vi "multiColorWormMolecule.vi"(0 "molecule":string) -> (1 "slider position":i32, 2 "filter wheel position":i32)   [LabVIEW 2017]
panel:
  # "Returns indexes of filter wheel and slider/shutter position\ngiven the molecule."
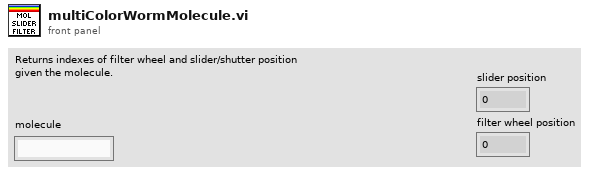
[diagram p1: front panel]
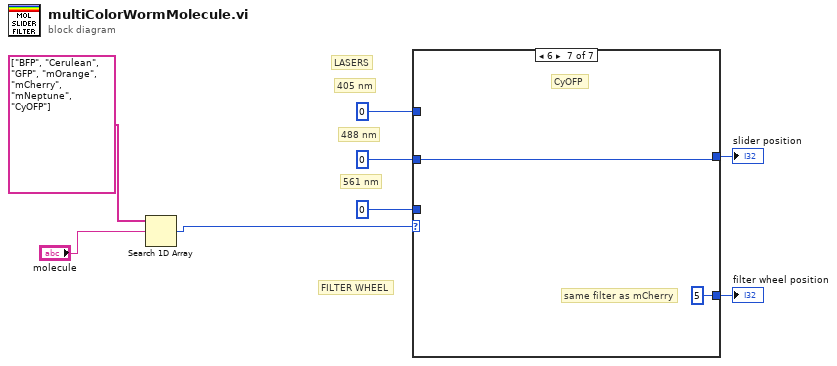
[diagram p0: block diagram]
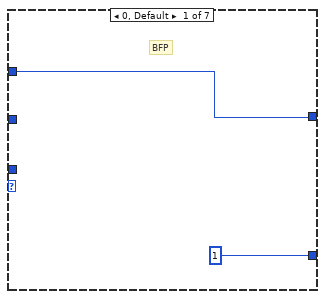
[diagram p2: hidden frame]
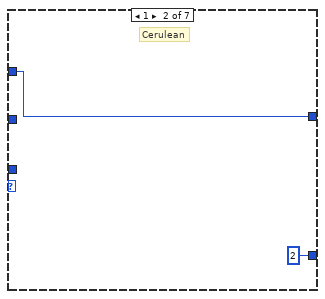
[diagram p3: hidden frame]
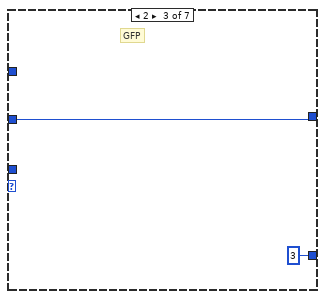
[diagram p4: hidden frame]
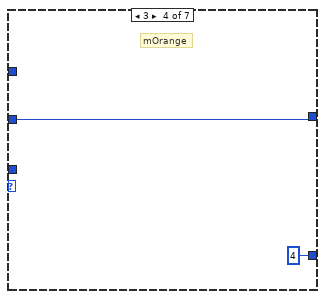
[diagram p5: hidden frame]
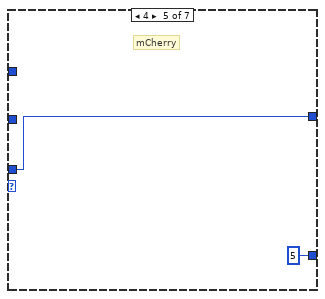
[diagram p6: hidden frame]
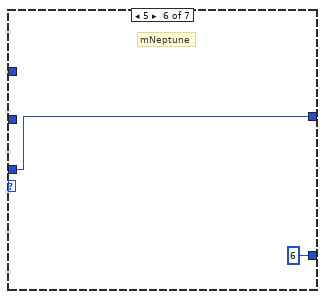
[diagram p7: hidden frame]
diagram:
  # "FILTER WHEEL"
  # "LASERS"
  # "561 nm"
  # "488 nm"
  # "405 nm"
  n1 = Search 1D Array(1D array=string[] ["BFP", "Cerulean", "GFP", "mOrange", "mCherry", "mNeptune", "CyOFP"], element="molecule") -> (index of element=w2:i32)  [unwired: 1 in]
  n2 = case shown="6" w2 {
    tunnel: 0 -> [w10 w12 _ _ _ _ _]
    tunnel: 0 -> [_ _ w14 w16 _ _ w21]
    tunnel: 0 -> [_ _ _ _ w17 w19 _]
    tunnel: [w10 w12 w14 w16 w17 w19 w21] -> w5
    tunnel: [1 2 3 4 5 6 5] -> w4
    frame 0, Default {
      # "BFP"
    }
    frame 1 {
      # "Cerulean"
    }
    frame 2 {
      # "GFP"
    }
    frame 3 {
      # "mOrange"
    }
    frame 4 {
      # "mCherry"
    }
    frame 5 {
      # "mNeptune"
    }
    frame 6 {
      # "same filter as mCherry"
      # "CyOFP"
    }
  }
  "slider position" <- w5
  "filter wheel position" <- w4
